vi "DATA_HORA_ALPHA_DELTA.vi"() -> (0 "SAIDA":string)   [LabVIEW 2018]
uses:
  Global_Telescopio.vi
panel:
  out "length":i32
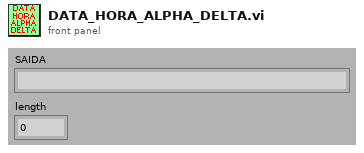
[diagram p1: front panel]
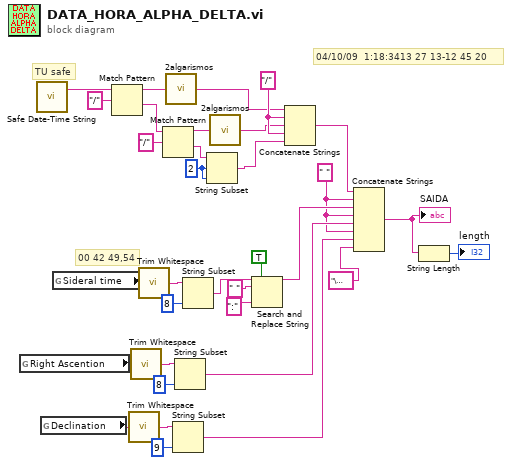
[diagram p0: block diagram]
diagram:
  w18 = "/"
  w19 = 2 ("offset (0)")
  w9 = " "
  # "TU safe"
  # "00 42 49,54"
  # "04/10/09  1:18:3413 27 13-12 45 20"
  n1 = global read "Global_Telescopio.vi" "Right Ascention"() -> (w11:string)
  n2 = call "Safe Date-Time String.vi"() -> ("Safe date string"=w1:string)  [unwired: 3 in, 1 out]
  n3 = global read "Global_Telescopio.vi" "Declination"() -> (w6:string)
  n4 = global read "Global_Telescopio.vi" "Sideral time"() -> (w33:string)
  n5 = Match Pattern(string=w1, regular expression="/") -> (before substring=w24:string, after substring=w22:string)  [unwired: 1 in, 2 out]
  n6 = call <vilib>:"Trim Whitespace.vi"("string"=w6) -> ("trimmed string"=w7:string)  [unwired: 1 in]
  n7 = call <vilib>:"Trim Whitespace.vi"("string"=w11) -> ("trimmed string"=w13:string)  [unwired: 1 in]
  n8 = call <vilib>:"Trim Whitespace.vi"("string"=w33) -> ("trimmed string"=w26:string)  [unwired: 1 in]
  n9 = Match Pattern(string=w22, regular expression="/") -> (before substring=w21:string, after substring=w20:string)  [unwired: 1 in, 2 out]
  n10 = call "2algarismos.vi"("entrada"=w24) -> ("saida"=w17:string)
  n11 = String Subset(string=w7, length (rest)=9 ("length (rest)")) -> (substring=w5:string)  [unwired: 1 in]
  n12 = String Subset(string=w13, length (rest)=8 ("length (rest)")) -> (substring=w10:string)  [unwired: 1 in]
  n13 = String Subset(string=w26, length (rest)=8 ("length (rest)")) -> (substring=w31:string)  [unwired: 1 in]
  n14 = String Subset(string=w20, offset (0)=w19, length (rest)=w19) -> (substring=w15:string)
  n15 = call "2algarismos.vi"("entrada"=w21) -> ("saida"=w16:string)
  n16 = Search and Replace String(replace all?=TRUE ("replace all? (F)"), input string=w31, search string=" ", replace string=":" ("replace string (\"\")")) -> (result string=w28:string)  [unwired: 4 in, 3 out]
  n17 = Concatenate Strings(w17, w18, w16, w18, w15) -> (w14:string)
  n18 = Concatenate Strings(w14, w9, w28, w9, w10, w9, w5, "\u0000") -> (w4:string)
  "SAIDA" <- w4
  n19 = String Length(string=w4) -> (length=→"length":i32)
